vi "Read Message.vi"(8 "error in (no error)":errorcluster, 11 "Simulated Detector in":refnum<class "Simulated Detector.lvclass">) -> (0 "error out":errorcluster, 2 "Message":string, 3 "Simulated Detector out":refnum<class "Simulated Detector.lvclass">)   [LabVIEW 2019, in "Simulated Detector.lvclass"]
uses:
  Simulated Detector.lvclass
  Simulated Detector.lvclass/Simulated Detector.ctl
  <vilib>/numeric/Random Number (Range) U64.vi
  <vilib>/numeric/sub_Random U32.vi
  <vilib>/Utility/error.llb/Error Cluster From Error Code.vi
  <vilib>/ErrorRing/Error Ring.xnode
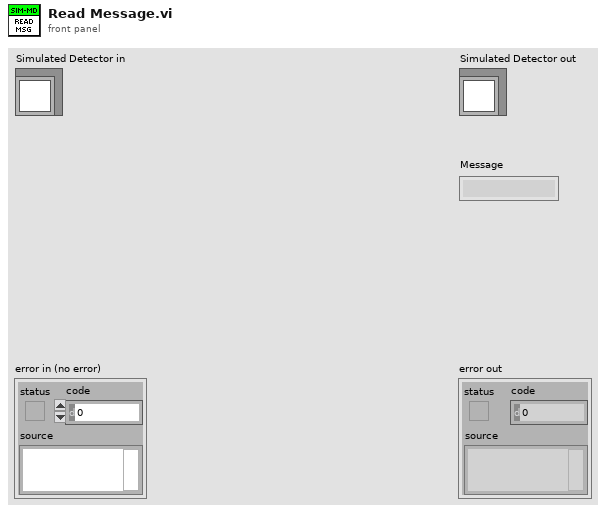
[diagram p1: front panel]
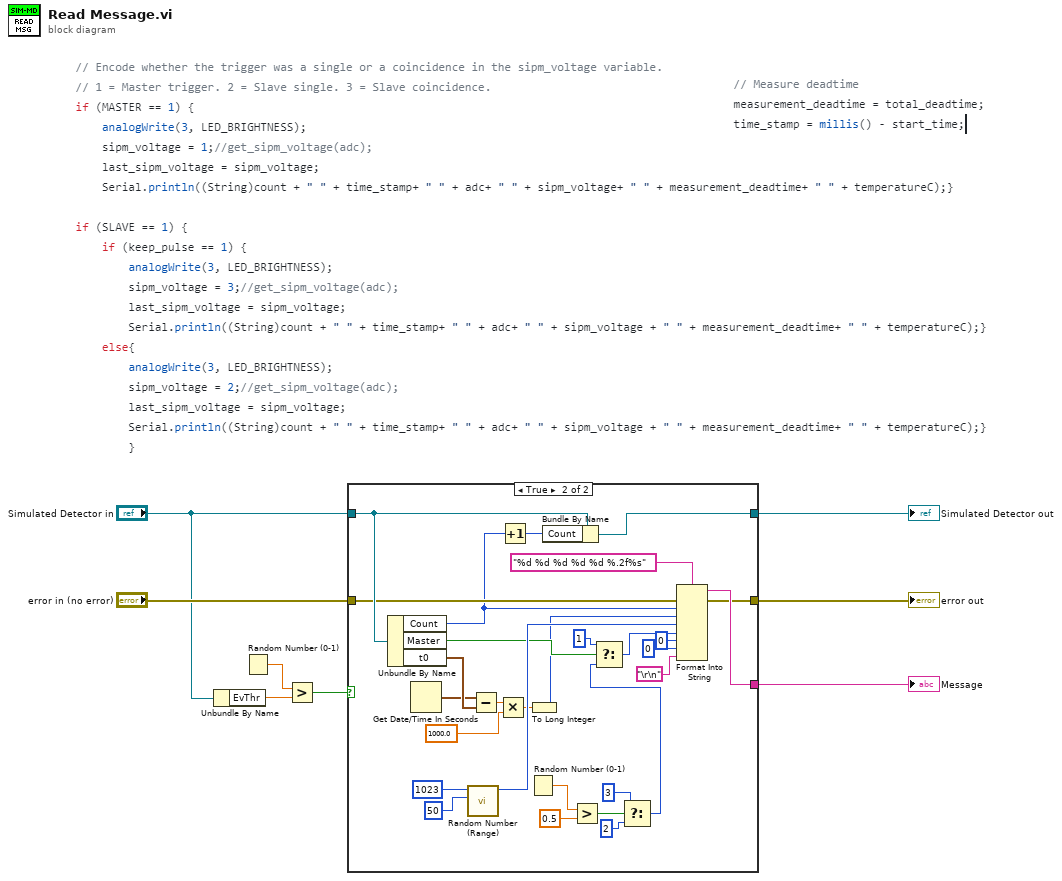
[diagram p0: block diagram]
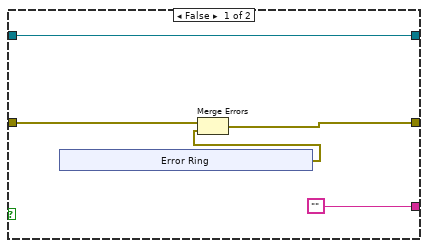
[diagram p2: hidden frame]
diagram:
  n1 = Unbundle By Name("Simulated Detector in") -> ("EvThr"=w1:dbl)
  n2 = Random Number (0-1)() -> (number: 0 to 1=w8:dbl)
  n3 = Greater?(x=w8, y=w1) -> (0:w7:bool)
  n4 = case shown="True" w7 {
    tunnel: ["" w46] -> w6
    tunnel: "Simulated Detector in" -> [w12 w45]
    tunnel: [w12 w41] -> w5
    tunnel: "error in (no error)" -> [w11 w44]
    tunnel: [w10 w43] -> w3
    frame False {
      n5 = xnode "Error Ring"() -> ("error out"=w9:errorcluster)
      n6 = Merge Errors(w11, w9) -> (w10:errorcluster)
    }
    frame True {
      n7 = Unbundle By Name(w45) -> ("Count"=w39:i32, "Master"=w35:bool, "t0"=w24:timestamp)
      n8 = Get Date/Time In Seconds() -> (seconds since 1Jan1904=w23:timestamp)
      n9 = call-poly <vilib>:"Random Number (Range).vi"("lower bound (0)"=u64 50, "upper bound (100)"=u64 1023) -> ("number"=w36:u64)  [unwired: 9 in]
      n10 = Subtract(x=w23, y=w24) -> (x-y=w22:dbl)
      n11 = Multiply(x=w22, y=1000.0 ("x")) -> (x*y=w19:dbl)
      n12 = Increment(x=w39) -> (x+1=w40:i32)
      n13 = Random Number (0-1)() -> (number: 0 to 1=w32:dbl)
      n14 = To Long Integer(number=w19) -> (32bit integer=w21:i32)
      n15 = Bundle By Name(cluster=w45, "Count"=w40) -> (w41:refnum<class "Simulated Detector.lvclass">)
      n16 = Greater?(x=w32, y=0.5) -> (0:w31:bool)
      n17 = Select(t=3, s=w31, f=2) -> (s? t:f=w30:i32)
      n18 = Select(t=1, s=w35, f=w30) -> (s? t:f=w27:i32)
      n19 = Format Into String(format string="%d %d %d %d %d %.2f%s", error in=w44, w39, w21, w36, w27, 0 ("input 5"), 0 ("input 6"), "\r\n") -> (resulting string=w46:string, error out=w43:errorcluster)  [unwired: 1 in]
    }
  }
  "error out" <- w3
  "Simulated Detector out" <- w5
  "Message" <- w6
